vi "Steering_converter.vi"(6 "Yaw":dbl, 9 "setpoint":dbl, 10 "output":dbl, 11 "Degree allowence":dbl) -> (3 "Steer":dbl)   [LabVIEW 2017]
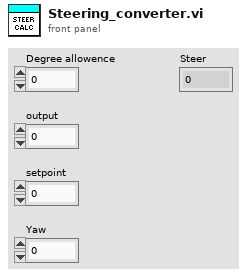
[diagram p1: front panel]
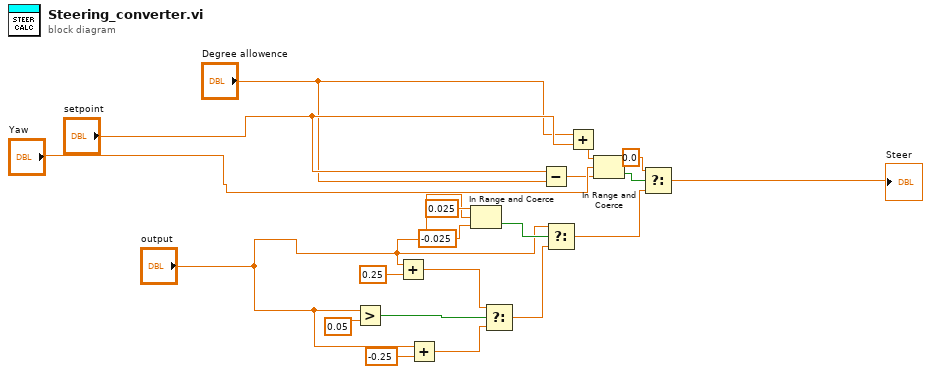
[diagram p0: block diagram]
diagram:
  n1 = Greater?(x="output", y=0.05) -> (0:w11:bool)
  n2 = Add(x="output", y=0.25) -> (x+y=w14:dbl)
  n3 = Add(x="output", y=-0.25) -> (x+y=w15:dbl)
  n4 = In Range and Coerce(upper limit=0.025, x="output", lower limit=-0.025) -> (In Range?=w10:bool)  [unwired: 1 out]
  n5 = Select(t=w14, s=w11, f=w15) -> (s? t:f=w17:dbl)
  n6 = Subtract(x="setpoint", y="Degree allowence") -> (x-y=w2:dbl)
  n7 = Select(t="output", s=w10, f=w17) -> (s? t:f=w18:dbl)
  n8 = Add(x="Degree allowence", y="setpoint") -> (x+y=w4:dbl)
  n9 = In Range and Coerce(upper limit=w4, x="Yaw", lower limit=w2) -> (In Range?=w5:bool)  [unwired: 1 out]
  n10 = Select(t=0.0, s=w5, f=w18) -> (s? t:f=→"Steer":dbl)
